vi "GearManipulatorOpen.vi"(8 "UpDownRefnum":string, 9 "OpenCloseRefnum":string, 10 "Gear Manipulator Open Close":enum16{"Open", "Close"}(ring), 11 "Gear Mainpulator Up Down":enum16{"Up", "Down"}(ring)) -> ()   [LabVIEW 2016, in "Gear Manipulator.lvclass"]
uses:
  Gear Manipulator.lvclass
  Gear Manipulator.lvclass/Gear Manipulator.ctl
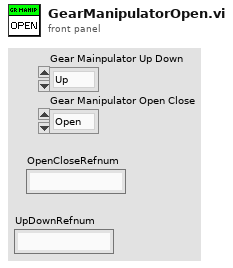
[diagram p1: front panel]
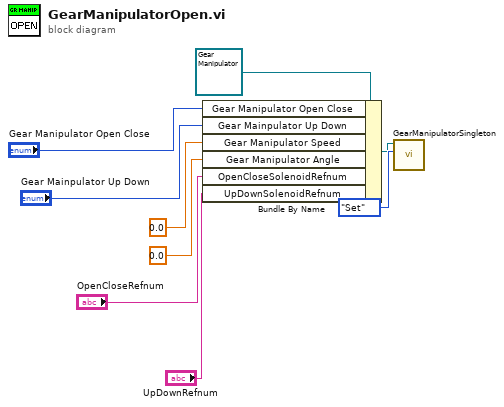
[diagram p0: block diagram]
diagram:
  n1 = Bundle By Name(cluster=refnum<class "Gear Manipulator.lvclass"> refnum ("Gear Manipulator.lvclass"), "Gear Manipulator Open Close"="Gear Manipulator Open Close", "Gear Mainpulator Up Down"="Gear Mainpulator Up Down", "Gear Manipulator Speed"=0.0, "Gear Manipulator Angle"=0.0, "OpenCloseSolenoidRefnum"="OpenCloseRefnum", "UpDownSolenoidRefnum"="UpDownRefnum") -> (w8:refnum<class "Gear Manipulator.lvclass">)
  n2 = call "GearManipulatorSingleton.vi"("Get/Set"=enum16{"Get", "Set"}."Set", "Gear Manipulator.lvclass"=w8) -> ()  [unwired: 8 in, 2 out]
